vi "Read Frequencies.vi"(8 "error in (no error)":errorcluster, 11 "Write Frequencies Msg in":refnum<class "Write Frequencies Msg.lvclass">) -> (0 "error out":errorcluster, 2 "Frequencies":dbl[](array[numeric]), 3 "Write Frequencies Msg out":refnum<class "Write Frequencies Msg.lvclass">)   [LabVIEW 2015, in "Write Frequencies Msg.lvclass"]
uses:
  Write Frequencies Msg.lvclass
  Write Frequencies Msg.lvclass/Write Frequencies Msg.ctl
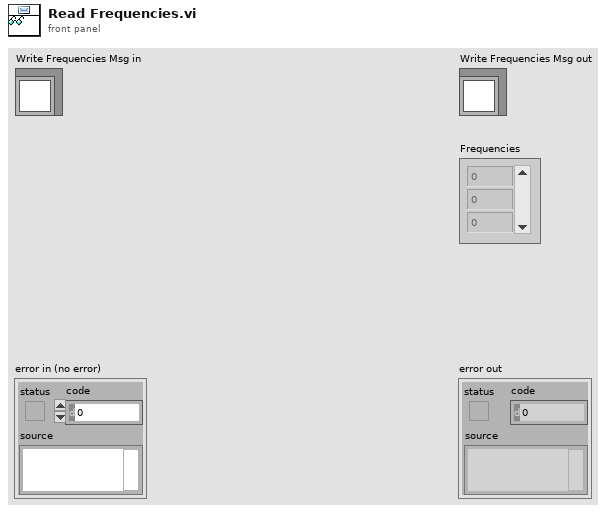
[diagram p1: front panel]
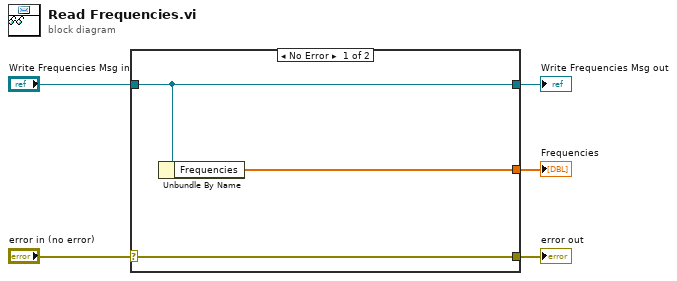
[diagram p0: block diagram]
diagram:
  n1 = case shown="No Error" "error in (no error)" {
    selector: "error in (no error)" -> [w8 w9]
    tunnel: [w8 w9] -> w4
    tunnel: [w7 w10] -> w2
    tunnel: "Write Frequencies Msg in" -> [w7 w10]
    tunnel: [w6 _] -> w1
    frame No Error {
      n2 = Unbundle By Name(w7) -> ("Frequencies"=w6:dbl[])
    }
    frame Error {
    }
  }
  "error out" <- w4
  "Write Frequencies Msg out" <- w2
  "Frequencies" <- w1
